vi "run_control.vi"() -> ()   [LabVIEW 2011]
uses:
  Dependencies/global.vi
panel:
  out "# of data":i32
  out "Real-time Data from Weather Station":string[][](array[string])
  out "Username":string
  out "Last Received Request":string
  in  "stop":bool
  out "Someone Connected?":bool
  out "Req / Res Error":errorcluster
  out "Remote Port":i64
  out "Remote Address":string
  out "Connection Error":errorcluster
  out "Real-time Data from PLCs (Actuation)":string[][](array[string])
  out "# of data":i32
  out "# of data":i32
  out "# of data":i32
  out "# of data":i32
  out "# of received data":u64
  out "Real-time Data from People Counter":string[][](array[string])
  out "Real-time Data from PLCs (Sensing)":string[][](array[string])
  out "Real-time Data from Motes":string[][](array[string])
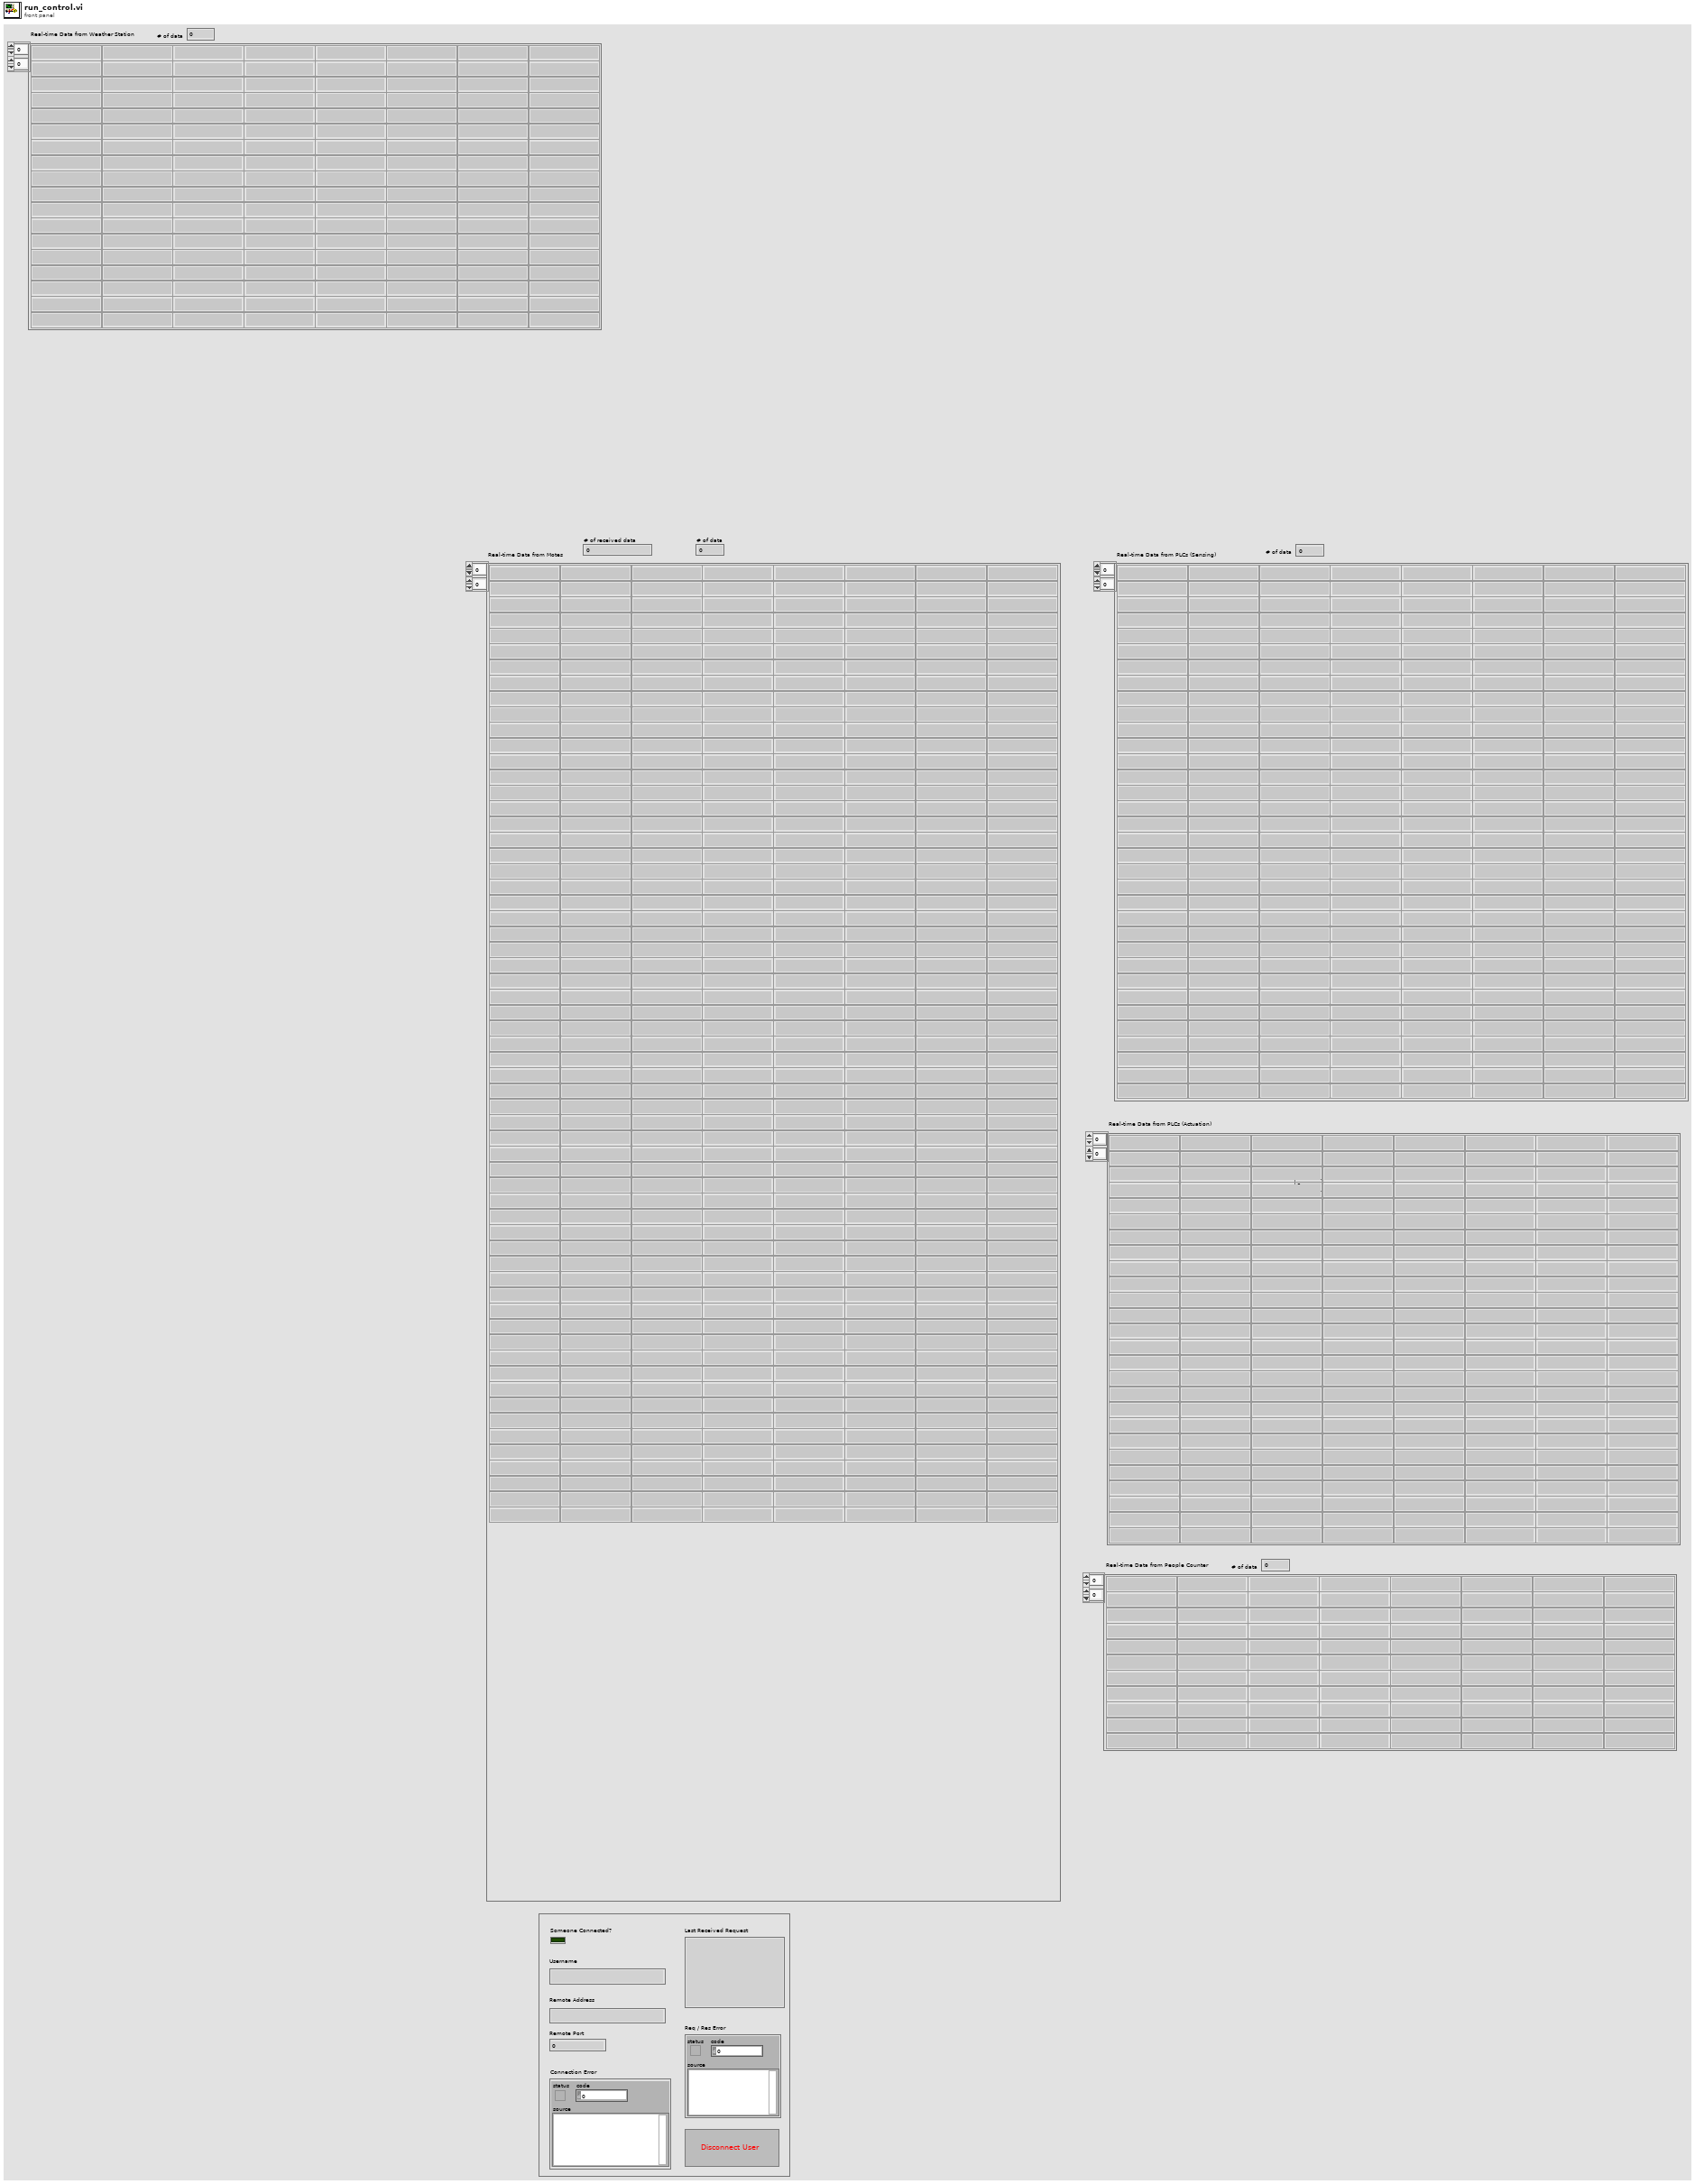
[diagram p1: front panel]
types:
  T1 = cluster{string, string, string, string, string, string, string, string}
  T2 = enum16{"Read", "Write", "ReadWrite", "BufferedRead", "BufferedReadWrite"}
  T3 = typedef "LVDateTimeRec.ctl" = cluster{"fractional second":dbl, "second":i32, "minute":i32, "hour":i32, "day of month":i32, "month":i32, "year":i32, "day of week":i32, "day of year":i32, "DST":i32}
  T4 = cluster{string, string, string, string, string, "date/time string":string, "output string":string, string}
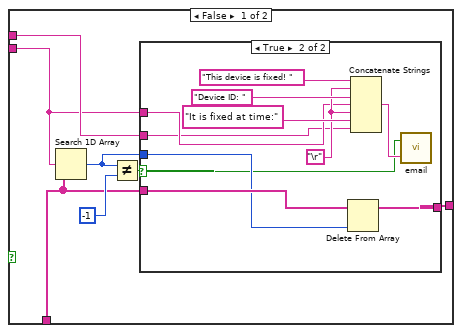
[diagram p3: hidden frame]
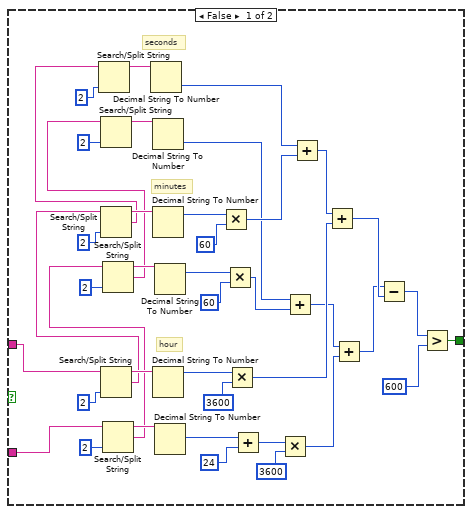
[diagram p6: hidden frame]
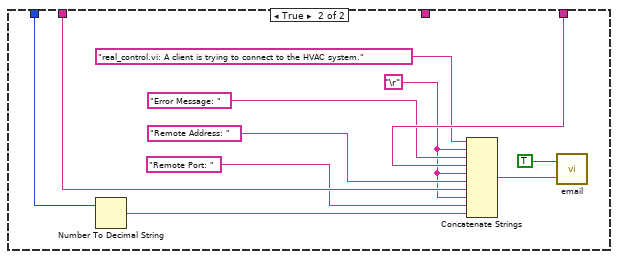
[diagram p7: hidden frame]
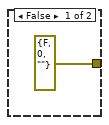
[diagram p8: hidden frame]
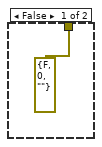
[diagram p9: hidden frame]
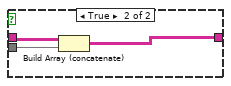
[diagram p10: hidden frame]
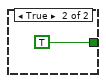
[diagram p11: hidden frame]
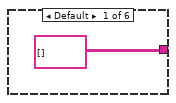
[diagram p12: hidden frame]
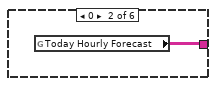
[diagram p13: hidden frame]
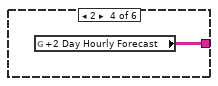
[diagram p14: hidden frame]
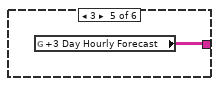
[diagram p15: hidden frame]
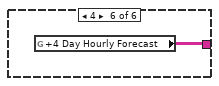
[diagram p16: hidden frame]
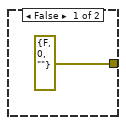
[diagram p17: hidden frame]
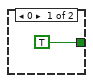
[diagram p18: hidden frame]
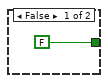
[diagram p19: hidden frame]
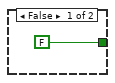
[diagram p20: hidden frame]
diagram:
  w1 = string[][] [["sourceType", "deviceID", "dataType", "signalID", "value", "timeStamp", "location", "coordinate"]] ("array")
  # "Real-time control Server"
  # "getting real-time data from database.vi"
  n1 = Bundle("", "", "", "", "", "", "", "") -> (w6:T1)  [unwired: 1 in]
  n2 = Obtain Queue(name (unnamed)="realtimeQue", element data type=w6) -> (queue out=w25:refnum<queue>)  [unwired: 3 in, 2 out]
  n3 = while {
    tunnel: w25 -> [w94]
    shift-right: [w41] -> _
    shift-left: w1 -> [w31]
    shift-right: [w40] -> _
    shift-left: w1 -> [w90]
    shift-right: [w79] -> _
    shift-left: w1 -> [w87]
    shift-right: [w42] -> _
    shift-left: w1 -> [w59]
    shift-right: [w29] -> _
    shift-left: w1 -> [w28]
    i -> [w86]
    stop <- TRUE continue-if-true
    n4 = Dequeue Element(queue=w94) -> (element=w44:T1)  [unwired: 2 in, 3 out]
    n5 = call "CommaToDot.vi"("Input"=w44) -> ("Output"=w30:T1)
    n6 = Unbundle(w30) -> (w33:string, w32:string, w27:string)  [unwired: 5 out]
    n7 = Unbundle(w30) -> (w55:string, w50:string, w49:string, w58:string)  [unwired: 4 out]
    n8 = Unbundle(w30) -> (w56:string, w52:string, w51:string)  [unwired: 5 out]
    n9 = Unbundle(w30) -> (w53:string, w46:string, w45:string)  [unwired: 5 out]
    n10 = Unbundle(w30) -> (w54:string, w48:string, w47:string, w57:string)  [unwired: 4 out]
    n11 = Equal?(x="6", y=w33) -> (x = y?=w39:bool)
    n12 = Not Equal?(x="A", y=w50) -> (x != y?=w71:bool)
    n13 = Equal?(x="2", y=w55) -> (x = y?=w70:bool)
    n14 = Equal?(x="A", y=w48) -> (x = y?=w66:bool)
    n15 = Equal?(x="2", y=w54) -> (x = y?=w67:bool)
    n16 = Equal?(x="1", y=w56) -> (x = y?=w92:bool)
    n17 = Equal?(x="3", y=w53) -> (x = y?=w89:bool)
    n18 = And(x=w71, y=w70) -> (x .and. y?=w69:bool)
    n19 = And(x=w66, y=w67) -> (x .and. y?=w68:bool)
    n20 = case shown="True" w39 {
      tunnel: w30 -> [_ w104]
      tunnel: w28 -> [w96 w98]
      tunnel: [w96 w99] -> w29
      tunnel: w32 -> [_ w103]
      tunnel: w27 -> [_ w97]
      frame False {
      }
      frame True {
        # "update array or add a new entry"
        # "search current array to see if the new data is already exists or not"
        n21 = for {
          tunnel: w98 -> [w116] mode=indexing
          tunnel: w103 -> [w119]
          tunnel: [w114] -> w102
          tunnel: [w118] -> w101
          tunnel: w97 -> [w115]
          i -> [w118]
          stop <- w114 stop-if-true
          # "key for weather station: deviceID and signalID"
          n22 = Index Array(array=w116, index=1) -> (element=w120:string)
          n23 = Equal?(x=w119, y=w120) -> (x = y?=w117:bool)
          n24 = case shown="True" w117 {
            tunnel: w116 -> [_ w126]
            tunnel: w115 -> [_ w124]
            tunnel: [FALSE w123] -> w114
            frame False {
            }
            frame True {
              n25 = Index Array(array=w126, index=3) -> (element=w125:string)
              n26 = Equal?(x=w124, y=w125) -> (x = y?=w123:bool)
            }
          }
        }
        n27 = Cluster To Array(cluster=w104) -> (array=w100:string[])
        n28 = case shown="True" w102 {
          tunnel: w98 -> [w109 w111]
          tunnel: w101 -> [w106 w110]
          tunnel: w100 -> [w108 w112]
          tunnel: [w107 w113] -> w99
          frame False {
            n29 = Increment(x=w106) -> (x+1=w105:i32)
            n30 = Insert Into Array(array=w109, index (row)=w105, new element=w108) -> (w107:string[][])  [unwired: 1 in]
          }
          frame True {
            n31 = Replace Array Subset(array=w111, new element=w112, index (row)=w110) -> (w113:string[][])  [unwired: 1 in]
          }
        }
      }
    }
    "Real-time Data from Weather Station" <- w29
    n32 = case shown="False" w69 {
      tunnel: w30 -> [_ w200]
      tunnel: w90 -> [w192 w195]
      tunnel: [w192 w196] -> w40
      tunnel: w49 -> [_ w194]
      tunnel: w58 -> [_ w193]
      frame False {
      }
      frame True {
        # "search current array to see if the new data is already exists or not"
        # "update array or add a new entry"
        n33 = for {
          tunnel: w195 -> [w211] mode=indexing
          tunnel: w194 -> [w215]
          tunnel: [w210] -> w199
          tunnel: [w214] -> w198
          tunnel: w193 -> [w212]
          i -> [w214]
          stop <- w210 stop-if-true
          # "key for plcs: signalID and location"
          n34 = Index Array(array=w211, index=3) -> (element=w216:string)
          n35 = Equal?(x=w215, y=w216) -> (x = y?=w213:bool)
          n36 = case shown="True" w213 {
            tunnel: w211 -> [_ w222]
            tunnel: w212 -> [_ w220]
            tunnel: [FALSE w219] -> w210
            frame False {
            }
            frame True {
              n37 = Index Array(array=w222, index=6) -> (element=w221:string)
              n38 = Equal?(x=w220, y=w221) -> (x = y?=w219:bool)
            }
          }
        }
        n39 = Cluster To Array(cluster=w200) -> (array=w197:string[])
        n40 = case shown="True" w199 {
          tunnel: w195 -> [w205 w207]
          tunnel: w198 -> [w202 w206]
          tunnel: w197 -> [w204 w208]
          tunnel: [w203 w209] -> w196
          frame False {
            n41 = Increment(x=w202) -> (x+1=w201:i32)
            n42 = Insert Into Array(array=w205, index (row)=w201, new element=w204) -> (w203:string[][])  [unwired: 1 in]
          }
          frame True {
            n43 = Replace Array Subset(array=w207, new element=w208, index (row)=w206) -> (w209:string[][])  [unwired: 1 in]
          }
        }
      }
    }
    "Real-time Data from PLCs (Sensing)" <- w40
    n44 = case shown="True" w92 {
      tunnel: w30 -> [_ w232]
      tunnel: w31 -> [w224 w226]
      tunnel: [w224 w227] -> w41
      tunnel: w52 -> [_ w231]
      tunnel: w51 -> [_ w225]
      frame False {
      }
      frame True {
        # "update array or add a new entry"
        # "search current array to see if the new data is already exists or not"
        n45 = for {
          tunnel: w226 -> [w244] mode=indexing
          tunnel: w231 -> [w247]
          tunnel: [w242] -> w230
          tunnel: [w246] -> w229
          tunnel: w225 -> [w243]
          i -> [w246]
          stop <- w242 stop-if-true
          # "key for motes: deviceID and dataType"
          n46 = Index Array(array=w244, index=1) -> (element=w248:string)
          n47 = Equal?(x=w247, y=w248) -> (x = y?=w245:bool)
          n48 = case shown="True" w245 {
            tunnel: w244 -> [_ w254]
            tunnel: w243 -> [_ w252]
            tunnel: [FALSE w251] -> w242
            frame False {
            }
            frame True {
              n49 = Index Array(array=w254, index=2) -> (element=w253:string)
              n50 = Equal?(x=w252, y=w253) -> (x = y?=w251:bool)
            }
          }
        }
        n51 = Cluster To Array(cluster=w232) -> (array=w228:string[])
        n52 = case shown="True" w230 {
          tunnel: w226 -> [w237 w239]
          tunnel: w229 -> [w234 w238]
          tunnel: w228 -> [w236 w240]
          tunnel: [w235 w241] -> w227
          frame False {
            n53 = Increment(x=w234) -> (x+1=w233:i32)
            n54 = Insert Into Array(array=w237, index (row)=w233, new element=w236) -> (w235:string[][])  [unwired: 1 in]
          }
          frame True {
            n55 = Replace Array Subset(array=w239, new element=w240, index (row)=w238) -> (w241:string[][])  [unwired: 1 in]
          }
        }
      }
    }
    "Real-time Data from Motes" <- w41
    n56 = case shown="True" w89 {
      tunnel: w30 -> [_ w168]
      tunnel: w87 -> [w160 w162]
      tunnel: [w160 w163] -> w79
      tunnel: w46 -> [_ w167]
      tunnel: w45 -> [_ w161]
      frame False {
      }
      frame True {
        # "update array or add a new entry"
        # "search current array to see if the new data is already exists or not"
        n57 = for {
          tunnel: w162 -> [w180] mode=indexing
          tunnel: w167 -> [w183]
          tunnel: [w178] -> w166
          tunnel: [w182] -> w165
          tunnel: w161 -> [w179]
          i -> [w182]
          stop <- w178 stop-if-true
          # "key for counter: deviceID and dataType"
          n58 = Index Array(array=w180, index=1) -> (element=w184:string)
          n59 = Equal?(x=w183, y=w184) -> (x = y?=w181:bool)
          n60 = case shown="True" w181 {
            tunnel: w180 -> [_ w190]
            tunnel: w179 -> [_ w188]
            tunnel: [FALSE w187] -> w178
            frame False {
            }
            frame True {
              n61 = Index Array(array=w190, index=2) -> (element=w189:string)
              n62 = Equal?(x=w188, y=w189) -> (x = y?=w187:bool)
            }
          }
        }
        n63 = Cluster To Array(cluster=w168) -> (array=w164:string[])
        n64 = case shown="True" w166 {
          tunnel: w162 -> [w173 w175]
          tunnel: w165 -> [w170 w174]
          tunnel: w164 -> [w172 w176]
          tunnel: [w171 w177] -> w163
          frame False {
            n65 = Increment(x=w170) -> (x+1=w169:i32)
            n66 = Insert Into Array(array=w173, index (row)=w169, new element=w172) -> (w171:string[][])  [unwired: 1 in]
          }
          frame True {
            n67 = Replace Array Subset(array=w175, new element=w176, index (row)=w174) -> (w177:string[][])  [unwired: 1 in]
          }
        }
      }
    }
    "Real-time Data from People Counter" <- w79
    n68 = case shown="True" w68 {
      tunnel: w30 -> [_ w136]
      tunnel: w59 -> [w128 w131]
      tunnel: [w128 w132] -> w42
      tunnel: w47 -> [_ w130]
      tunnel: w57 -> [_ w129]
      frame False {
      }
      frame True {
        # "search current array to see if the new data is already exists or not"
        # "update array or add a new entry"
        n69 = for {
          tunnel: w131 -> [w147] mode=indexing
          tunnel: w130 -> [w151]
          tunnel: [w146] -> w135
          tunnel: [w150] -> w134
          tunnel: w129 -> [w148]
          i -> [w150]
          stop <- w146 stop-if-true
          # "key for plcs: signalID and location"
          n70 = Index Array(array=w147, index=3) -> (element=w152:string)
          n71 = Equal?(x=w151, y=w152) -> (x = y?=w149:bool)
          n72 = case shown="True" w149 {
            tunnel: w147 -> [_ w158]
            tunnel: w148 -> [_ w156]
            tunnel: [FALSE w155] -> w146
            frame False {
            }
            frame True {
              n73 = Index Array(array=w158, index=6) -> (element=w157:string)
              n74 = Equal?(x=w156, y=w157) -> (x = y?=w155:bool)
            }
          }
        }
        n75 = Cluster To Array(cluster=w136) -> (array=w133:string[])
        n76 = case shown="False" w135 {
          tunnel: w131 -> [w141 w143]
          tunnel: w134 -> [w138 w142]
          tunnel: w133 -> [w140 w144]
          tunnel: [w139 w145] -> w132
          frame False {
            n77 = Increment(x=w138) -> (x+1=w137:i32)
            n78 = Insert Into Array(array=w141, index (row)=w137, new element=w140) -> (w139:string[][])  [unwired: 1 in]
          }
          frame True {
            n79 = Replace Array Subset(array=w143, new element=w144, index (row)=w142) -> (w145:string[][])  [unwired: 1 in]
          }
        }
      }
    }
    "Real-time Data from PLCs (Actuation)" <- w42
    n80 = Array Size(array=w29) -> (size(s)=w36:i32[])
    n81 = Array Size(array=w79) -> (size(s)=w80:i32[])
    n82 = Array Size(array=w41) -> (size(s)=w82:i32[])
    n83 = global write "global.vi" "Motes"(w41) -> ()
    n84 = global write "global.vi" "PLC Sensing"(w40) -> ()
    n85 = Array Size(array=w40) -> (size(s)=w85:i32[])
    n86 = Array Size(array=w42) -> (size(s)=w61:i32[])
    n87 = Index Array(array=w40, index (row)=1) -> ()  [unwired: 1 in, 1 out]
    n88 = global write "global.vi" "Actuation PLC"(w42) -> ()
    n89 = Index Array(array=w36, index=0) -> (element=w35:i32)
    n90 = Index Array(array=w80, index=0) -> (element=w74:i32)
    n91 = Index Array(array=w82, index=0) -> (element=w78:i32)
    n92 = Index Array(array=w85, index=0) -> (element=w76:i32)
    n93 = Index Array(array=w61, index=0) -> (element=w63:i32)
    n94 = Decrement(x=w35) -> (x-1=→"# of data":i32)
    n95 = Decrement(x=w78) -> (x-1=→"# of data":i32)
    n96 = Decrement(x=w74) -> (x-1=→"# of data":i32)
    n97 = Decrement(x=w76) -> (x-1=→"# of data":i32)
    n98 = Decrement(x=w63) -> (x-1=→"# of data":i32)
    "# of received data" <- w86
  }
  n99 = while {
    i -> [w258]
    stop <- TRUE continue-if-true
    n100 = local read "Real-time Data from PLCs (Actuation)"() -> (w257:string[][])
    n101 = local read "Real-time Data from Weather Station"() -> (w256:string[][])
    n102 = local read "Real-time Data from Motes"() -> (w260:string[][])
    n103 = call "writegraph.vi"("FromWeatherStation"=w256, "FromPLC"=w257, "Numeric"=w258, "FromMotes"=w260) -> ()  [unwired: 2 in]
    n104 = Wait (ms)(milliseconds to wait=u32 60000) -> ()  [unwired: 1 out]
  }
  n105 = Wait (ms)(milliseconds to wait=u32 30000) -> (millisecond timer value=w2:u32)
  n106 = flat-sequence {
    tunnel: w2 -> [_]
    frame #0 {
      n107 = while {
        shift-right: [w264] -> _
        shift-left: string[] [] ("Array") -> [w265]
        stop <- TRUE continue-if-true
        n108 = local read "# of data"() -> (w263:i32)
        n109 = Format Date/Time String(time format string (%c)="%y%m%d%H%M%S") -> (date/time string=w266:string)  [unwired: 2 in]
        n110 = for {
          N: w263 -> [_]
          tunnel: w266 -> [w288]
          shift-right: [w270] -> w264
          shift-left: w265 -> [w271]
          i -> [w296]
          # "same month?"
          # "same year?"
          n111 = Increment(x=w296) -> (x+1=w295:i32)
          n112 = Search/Split String(string=w288, offset (0)=2) -> (substring before match=w290:string, match + rest of string=w281:string)  [unwired: 1 in, 1 out]
          n113 = Search/Split String(string=w281, offset (0)=2) -> (substring before match=w283:string, match + rest of string=w274:string)  [unwired: 1 in, 1 out]
          n114 = local read "Real-time Data from Motes"() -> (w294:string[][])
          n115 = Decimal String To Number(string=w283) -> (number=w279:i32)  [unwired: 2 in, 1 out]
          n116 = Decimal String To Number(string=w290) -> (number=w289:i32)  [unwired: 2 in, 1 out]
          n117 = Index Array(array=w294, index (row)=w295, index (col)=1 ("disabled index (col)")) -> (element=w272:string)
          n118 = Index Array(array=w294, index (row)=w295, index (col)=5 ("disabled index (col)")) -> (element=w273:string)
          n119 = Search/Split String(string=w273, offset (0)=2) -> (substring before match=w292:string, match + rest of string=w282:string)  [unwired: 1 in, 1 out]
          n120 = Search/Split String(string=w282, offset (0)=2) -> (substring before match=w285:string, match + rest of string=w275:string)  [unwired: 1 in, 1 out]
          n121 = Decimal String To Number(string=w285) -> (number=w280:i32)  [unwired: 2 in, 1 out]
          n122 = Decimal String To Number(string=w292) -> (number=w287:i32)  [unwired: 2 in, 1 out]
          n123 = Equal?(x=w280, y=w279) -> (x = y?=w278:bool)
          n124 = Equal?(x=w287, y=w289) -> (x = y?=w277:bool)
          n125 = And(x=w277, y=w278) -> (x .and. y?=w276:bool)
          n126 = case shown="True" w276 {
            tunnel: w275 -> [_ w311]
            tunnel: w274 -> [_ w310]
            tunnel: w273 -> [_ w303]
            tunnel: w272 -> [_ w302]
            tunnel: w271 -> [w299 w301]
            tunnel: [w299 w300] -> w270
            frame False {
            }
            frame True {
              # "same day?"
              n127 = Search/Split String(string=w311, offset (0)=2) -> (substring before match=w314:string, match + rest of string=w306:string)  [unwired: 1 in, 1 out]
              n128 = Search/Split String(string=w310, offset (0)=2) -> (substring before match=w312:string, match + rest of string=w305:string)  [unwired: 1 in, 1 out]
              n129 = Decimal String To Number(string=w314) -> (number=w309:i32)  [unwired: 2 in, 1 out]
              n130 = Decimal String To Number(string=w312) -> (number=w308:i32)  [unwired: 2 in, 1 out]
              n131 = Equal?(x=w309, y=w308) -> (x = y?=w307:bool)
              n132 = case shown="True" w307 {
                tunnel: w306 -> [w357 w426]
                tunnel: w305 -> [w356 w425]
                tunnel: [w351 w392] -> w304
                frame False {
                  # "hour"
                  # "minutes"
                  # "seconds"
                  n133 = Search/Split String(string=w357, offset (0)=2) -> (substring before match=w390:string, match + rest of string=w383:string)  [unwired: 1 in, 1 out]
                  n134 = Search/Split String(string=w383, offset (0)=2) -> (substring before match=w386:string, match + rest of string=w377:string)  [unwired: 1 in, 1 out]
                  n135 = Search/Split String(string=w377, offset (0)=2) -> (substring before match=w380:string)  [unwired: 1 in, 2 out]
                  n136 = Search/Split String(string=w356, offset (0)=2) -> (substring before match=w388:string, match + rest of string=w382:string)  [unwired: 1 in, 1 out]
                  n137 = Search/Split String(string=w382, offset (0)=2) -> (substring before match=w384:string, match + rest of string=w376:string)  [unwired: 1 in, 1 out]
                  n138 = Search/Split String(string=w376, offset (0)=2) -> (substring before match=w378:string)  [unwired: 1 in, 2 out]
                  n139 = Decimal String To Number(string=w380) -> (number=w368:i32)  [unwired: 2 in, 1 out]
                  n140 = Decimal String To Number(string=w378) -> (number=w364:i32)  [unwired: 2 in, 1 out]
                  n141 = Decimal String To Number(string=w386) -> (number=w375:i32)  [unwired: 2 in, 1 out]
                  n142 = Decimal String To Number(string=w390) -> (number=w370:i32)  [unwired: 2 in, 1 out]
                  n143 = Decimal String To Number(string=w384) -> (number=w372:i32)  [unwired: 2 in, 1 out]
                  n144 = Decimal String To Number(string=w388) -> (number=w354:i32)  [unwired: 2 in, 1 out]
                  n145 = Multiply(x=w375, y=60) -> (x*y=w367:i32)
                  n146 = Multiply(x=w372, y=60) -> (x*y=w363:i32)
                  n147 = Multiply(x=w370, y=3600) -> (x*y=w365:i32)
                  n148 = Add(x=w354, y=24) -> (x+y=w353:i32)
                  n149 = Multiply(x=w353, y=3600) -> (x*y=w352:i32)
                  n150 = Add(x=w364, y=w363) -> (x+y=w362:i32)
                  n151 = Add(x=w368, y=w367) -> (x+y=w366:i32)
                  n152 = Add(x=w366, y=w365) -> (x+y=w361:i32)
                  n153 = Add(x=w362, y=w352) -> (x+y=w360:i32)
                  n154 = Subtract(x=w360, y=w361) -> (x-y=w359:i32)
                  n155 = Greater?(x=w359, y=600) -> (0:w351:bool)
                }
                frame True {
                  # "hour"
                  # "minutes"
                  # "seconds"
                  n156 = Search/Split String(string=w426, offset (0)=2) -> (substring before match=w429:string, match + rest of string=w420:string)  [unwired: 1 in, 1 out]
                  n157 = Search/Split String(string=w420, offset (0)=2) -> (substring before match=w423:string, match + rest of string=w414:string)  [unwired: 1 in, 1 out]
                  n158 = Search/Split String(string=w414, offset (0)=2) -> (substring before match=w417:string)  [unwired: 1 in, 2 out]
                  n159 = Search/Split String(string=w425, offset (0)=2) -> (substring before match=w427:string, match + rest of string=w419:string)  [unwired: 1 in, 1 out]
                  n160 = Search/Split String(string=w419, offset (0)=2) -> (substring before match=w421:string, match + rest of string=w413:string)  [unwired: 1 in, 1 out]
                  n161 = Search/Split String(string=w413, offset (0)=2) -> (substring before match=w415:string)  [unwired: 1 in, 2 out]
                  n162 = Decimal String To Number(string=w417) -> (number=w404:i32)  [unwired: 2 in, 1 out]
                  n163 = Decimal String To Number(string=w415) -> (number=w400:i32)  [unwired: 2 in, 1 out]
                  n164 = Decimal String To Number(string=w423) -> (number=w412:i32)  [unwired: 2 in, 1 out]
                  n165 = Decimal String To Number(string=w429) -> (number=w407:i32)  [unwired: 2 in, 1 out]
                  n166 = Decimal String To Number(string=w421) -> (number=w409:i32)  [unwired: 2 in, 1 out]
                  n167 = Decimal String To Number(string=w427) -> (number=w405:i32)  [unwired: 2 in, 1 out]
                  n168 = Multiply(x=w412, y=60) -> (x*y=w403:i32)
                  n169 = Multiply(x=w409, y=60) -> (x*y=w399:i32)
                  n170 = Multiply(x=w407, y=3600) -> (x*y=w401:i32)
                  n171 = Multiply(x=w405, y=3600) -> (x*y=w397:i32)
                  n172 = Add(x=w400, y=w399) -> (x+y=w398:i32)
                  n173 = Add(x=w404, y=w403) -> (x+y=w402:i32)
                  n174 = Add(x=w402, y=w401) -> (x+y=w396:i32)
                  n175 = Add(x=w398, y=w397) -> (x+y=w395:i32)
                  n176 = Subtract(x=w395, y=w396) -> (x-y=w394:i32)
                  n177 = Greater?(x=w394, y=600) -> (0:w392:bool)
                }
              }
              n178 = case shown="True" w304 {
                tunnel: w302 -> [w316 w335]
                tunnel: w303 -> [w317 w339]
                tunnel: w301 -> [w320 w338]
                tunnel: [w318 w337] -> w300
                frame False {
                  n179 = Search 1D Array(1D array=w320, element=w316) -> (index of element=w319:i32)  [unwired: 1 in]
                  n180 = Not Equal?(x=w319, y=-1) -> (x != y?=w321:bool)
                  n181 = case shown="True" w321 {
                    selector: w321 -> [_ w326]
                    tunnel: w320 -> [w323 w334]
                    tunnel: w319 -> [_ w329]
                    tunnel: [w323 w333] -> w318
                    tunnel: w316 -> [_ w325]
                    tunnel: w317 -> [_ w324]
                    frame False {
                    }
                    frame True {
                      w328 = "\r"
                      n182 = Delete From Array(array=w334, index=w329) -> (array with subset deleted=w333:string[])  [unwired: 1 in, 1 out]
                      n183 = Concatenate Strings("This device is fixed! " ("string"), w328, "Device ID: " ("string"), w325, w328, "It is fixed at time:" ("string"), w324) -> (w327:string)
                      n184 = call "email.vi"("Body"=w327, "Enable"=w326) -> ()  [unwired: 1 in]
                    }
                  }
                }
                frame True {
                  w344 = "\r"
                  n185 = Search 1D Array(1D array=w338, element=w335) -> (index of element=w341:i32)  [unwired: 1 in]
                  n186 = Equal?(x=w341, y=-1) -> (x = y?=w336:bool)
                  n187 = case shown="True" w336 {
                    tunnel: w338 -> [w347 w350]
                    tunnel: [w347 w349] -> w337
                    tunnel: w335 -> [_ w348]
                    frame False {
                    }
                    frame True {
                      n188 = Insert Into Array(array=w350, new element=w348) -> (w349:string[])  [unwired: 1 in]
                    }
                  }
                  n189 = Concatenate Strings("This device is not working! " ("string"), w344, "Device ID: " ("string"), w335, w344, "No data received from this mote since time:" ("string"), w339) -> (w342:string)
                  n190 = call "email.vi"("Body"=w342, "Enable"=w336) -> ()  [unwired: 1 in]
                }
              }
            }
          }
        }
        n191 = Wait (ms)(milliseconds to wait=u32 30000) -> ()  [unwired: 1 out]
      }
    }
  }
  n192 = Bundle("", "", "", "", "", "", "", "") -> (w20:T1)  [unwired: 1 in]
  n193 = Obtain Queue(max queue size (-1, unlimited)=-1, name (unnamed)="databaseQue", element data type=w20) -> (queue out=w15:refnum<queue>)  [unwired: 2 in, 2 out]
  n194 = while {
    tunnel: w15 -> [w439]
    stop <- TRUE continue-if-true
    n195 = call <vilib>:"TCP Listen.vi"("port"=u16 6342) -> ("error out"=w434:errorcluster, "remote port"=w432:u16, "remote address"=w433:string, "connection ID"=w435:refnum<k5>)  [unwired: 6 in, 1 out]
    "Remote Address" <- w433
    "Remote Port" <- w432
    n196 = local write "Someone Connected?"(FALSE ("Someone Connected?")) -> ()
    n197 = call "credentialCheck.vi"("connection ID in"=w435, "error in"=w434) -> ("connection ID out"=w442:refnum<k5>, "user"=w437:string, "error out"=w441:errorcluster)
    "Connection Error" <- w441
    "Username" <- w437
    n198 = Unbundle(w441) -> ("status"=w438:bool, "source"=w440:string)  [unwired: 1 out]
    n199 = case shown="False" w438 {
      tunnel: w432 -> [w445 w463]
      tunnel: w440 -> [_ w462]
      tunnel: w433 -> [w446 w458]
      tunnel: w437 -> [w444 _]
      frame False {
        w449 = "\r"
        n200 = Number To Decimal String(number=w445) -> (decimal integer string=w447:string)  [unwired: 1 in]
        n201 = Concatenate Strings("real_control.vi: A client connected to the HVAC system.", w449, "Username: ", w444, w449, "Remote Address: ", w446, w449, "Remote Port: ", w447) -> (w454:string)
        n202 = call "email.vi"("Body"=w454, "Enable"=FALSE) -> ()  [unwired: 1 in]
      }
      frame True {
        w457 = "\r"
        n203 = Number To Decimal String(number=w463) -> (decimal integer string=w455:string)  [unwired: 1 in]
        n204 = Concatenate Strings("real_control.vi: A client is trying to connect to the HVAC system.", w457, "Error Message: ", w462, w457, "Remote Address: ", w458, w457, "Remote Port: ", w455) -> (w465:string)
        n205 = call "email.vi"("Body"=w465, "Enable"=TRUE) -> ()  [unwired: 1 in]
      }
    }
    n206 = case shown="No Error" w441 {
      tunnel: w442 -> [w467 _]
      tunnel: w439 -> [w466 _]
      frame No Error {
        n207 = while {
          tunnel: w467 -> [w536]
          tunnel: w466 -> [w493]
          stop <- w475 stop-if-true
          # "signalID"
          # "To hour"
          # "From hour"
          # "signalID"
          # "deviceID"
          # "dataType"
          # "data"
          # "stop the loop if any problem\noccures in the TCP blocks. Normally\nit means the client terminated the\nconnection."
          # "location"
          # "signalID"
          # "dataType"
          # "deviceID"
          # "Then read all input \nparameters from client"
          # "signalID"
          # "dataType"
          # "deviceID"
          # "first read the size of input \nparameters from client"
          n208 = TCP Read(connection ID=w536, bytes to read=10, 9:-1 ("timeout ms (25000)")) -> (connection ID out=w532:refnum<k5>, data out=w533:string, error out=w531:errorcluster)  [unwired: 2 in]
          n209 = local write "Someone Connected?"(TRUE ("Someone Connected?")) -> ()
          n210 = Decimal String To Number(string=w533) -> (number=w530:i32)  [unwired: 2 in, 1 out]
          n211 = TCP Read(connection ID=w532, bytes to read=w530, error in (no error)=w531) -> (connection ID out=w479:refnum<k5>, data out=w470:string, error out=w523:errorcluster)  [unwired: 2 in]
          "Last Received Request" <- w470
          n212 = Pick Line(multi-line string=w470, line index=2) -> (output string=w503:string)  [unwired: 1 in]
          n213 = Pick Line(multi-line string=w470, line index=1) -> (output string=w502:string)  [unwired: 1 in]
          n214 = Pick Line(multi-line string=w470, line index=3) -> (output string=w504:string)  [unwired: 1 in]
          n215 = Pick Line(multi-line string=w470, line index=0) -> (output string=w501:string)  [unwired: 1 in]
          n216 = Pick Line(multi-line string=w470, line index=0) -> (output string=w482:string)  [unwired: 1 in]
          n217 = Pick Line(multi-line string=w470, line index=1) -> (output string=w485:string)  [unwired: 1 in]
          n218 = Pick Line(multi-line string=w470, line index=0) -> (output string=w487:string)  [unwired: 1 in]
          n219 = Pick Line(multi-line string=w470, line index=2) -> (output string=w484:string)  [unwired: 1 in]
          n220 = Pick Line(multi-line string=w470, line index=2) -> (output string=w508:string)  [unwired: 1 in]
          n221 = Pick Line(multi-line string=w470, line index=1) -> (output string=w476:string)  [unwired: 1 in]
          n222 = Pick Line(multi-line string=w470, line index=3) -> (output string=w506:string)  [unwired: 1 in]
          n223 = Pick Line(multi-line string=w470, line index=0) -> (output string=w509:string)  [unwired: 1 in]
          n224 = Pick Line(multi-line string=w470, line index=2) -> (output string=w471:string)  [unwired: 1 in]
          n225 = Pick Line(multi-line string=w470, line index=1) -> (output string=w522:string)  [unwired: 1 in]
          n226 = Pick Line(multi-line string=w470, line index=3) -> (output string=w469:string)  [unwired: 1 in]
          n227 = Pick Line(multi-line string=w470, line index=0) -> (output string=w521:string)  [unwired: 1 in]
          n228 = Pick Line(multi-line string=w470, line index=2) -> (output string=w526:string)  [unwired: 1 in]
          n229 = Pick Line(multi-line string=w470, line index=1) -> (output string=w527:string)  [unwired: 1 in]
          n230 = Pick Line(multi-line string=w470, line index=3) -> (output string=w525:string)  [unwired: 1 in]
          n231 = Pick Line(multi-line string=w470, line index=0) -> (output string=w528:string)  [unwired: 1 in]
          n232 = Equal?(x="GetDataWeatherNow", y=w482) -> (x = y?=w483:bool)
          n233 = Equal?(x="GetDataPCounter", y=w501) -> (x = y?=w499:bool)
          n234 = Equal?(x="GetDataWeatherForecast", y=w487) -> (x = y?=w486:bool)
          n235 = Equal?(x="GetDataPlcs", y=w521) -> (x = y?=w519:bool)
          n236 = case shown="True" w499 {
            tunnel: w502 -> [_ w655]
            tunnel: w503 -> [_ w654]
            tunnel: w504 -> [_ w653]
            tunnel: w479 -> [_ w647]
            tunnel: [errorcluster {"status"=FALSE, "code"=0, "source"=""} ("error IO") w648] -> w494
            frame False {
            }
            frame True {
              # "check each row of the array to see if it matches. If yes, append that row to the result array"
              n237 = local read "Real-time Data from People Counter"() -> (w650:string[][])
              n238 = for {
                tunnel: w650 -> [w681] mode=indexing
                tunnel: w655 -> [w683]
                tunnel: w654 -> [w688]
                tunnel: w653 -> [w687]
                shift-right: [w685] -> w651
                shift-left: string[][] [] -> [w682]
                i -> [w680]
                stop <- TRUE continue-if-true
                n239 = case shown="Default" w680 {
                  tunnel: w688 -> [_ w698]
                  tunnel: w687 -> [_ w697]
                  tunnel: [TRUE w696] -> w686
                  tunnel: w683 -> [_ w695]
                  tunnel: w681 -> [_ w690]
                  frame 0 {
                  }
                  frame Default {
                    n240 = Index Array(array=w690, index=1) -> (element=w699:string)
                    n241 = Empty String/Path?(string/path=w695) -> (empty?=w693:bool)
                    n242 = Equal?(x=w695, y=w699) -> (x = y?=w694:bool)
                    n243 = Or(x=w693, y=w694) -> (x .or. y?=w692:bool)
                    n244 = case shown="True" w692 {
                      tunnel: w690 -> [_ w715]
                      tunnel: w698 -> [_ w710]
                      tunnel: [FALSE w713] -> w691
                      frame False {
                      }
                      frame True {
                        n245 = Index Array(array=w715, index=2) -> (element=w714:string)
                        n246 = Empty String/Path?(string/path=w710) -> (empty?=w711:bool)
                        n247 = Equal?(x=w710, y=w714) -> (x = y?=w712:bool)
                        n248 = Or(x=w711, y=w712) -> (x .or. y?=w713:bool)
                      }
                    }
                    n249 = case shown="True" w691 {
                      tunnel: w690 -> [_ w707]
                      tunnel: w697 -> [_ w703]
                      tunnel: [FALSE w702] -> w696
                      frame False {
                      }
                      frame True {
                        n250 = Index Array(array=w707, index=3) -> (element=w706:string)
                        n251 = Equal?(x=w703, y=w706) -> (x = y?=w705:bool)
                        n252 = Empty String/Path?(string/path=w703) -> (empty?=w704:bool)
                        n253 = Or(x=w704, y=w705) -> (x .or. y?=w702:bool)
                      }
                    }
                  }
                }
                n254 = case shown="True" w686 {
                  tunnel: w682 -> [w717 w720]
                  tunnel: w681 -> [_ w719]
                  tunnel: [w717 w718] -> w685
                  frame False {
                  }
                  frame True {
                    n255 = Build Array (concatenate)(w720, w719) -> (w718:string[][])
                  }
                }
              }
              n256 = flat-sequence {
                tunnel: w651 -> [w658]
                tunnel: w647 -> [w657]
                tunnel: [w656] -> w649
                tunnel: w649 -> [w672]
                tunnel: [w671] -> w648
                tunnel: w647 -> [w670]
                frame #0 {
                  # "send each element of the array through the TCP connection"
                  n257 = for {
                    tunnel: w658 -> [w661] mode=indexing
                    tunnel: w657 -> [w660]
                    tunnel: [w659] -> w656
                    n258 = for {
                      tunnel: w661 -> [w664] mode=indexing
                      tunnel: w660 -> [w663]
                      tunnel: [w662] -> w659
                      n259 = String Length(string=w664) -> (length=w668:i32)
                      n260 = Number To Decimal String(number=w668, width (-)=i16 10) -> (decimal integer string=w667:string)
                      n261 = TCP Write(connection ID=w663, data in=w667) -> (connection ID out=w665:refnum<k5>, error out=w666:errorcluster)  [unwired: 2 in, 1 out]
                      n262 = TCP Write(connection ID=w665, data in=w664, error in (no error)=w666) -> (error out=w662:errorcluster)  [unwired: 1 in, 2 out]
                    }
                  }
                }
                frame #1 {
                  w674 = "EndOfTx" ("data in")
                  n263 = String Length(string=w674) -> (length=w677:i32)
                  n264 = Number To Decimal String(number=w677, width (-)=i16 10) -> (decimal integer string=w678:string)
                  n265 = TCP Write(connection ID=w670, data in=w678) -> (connection ID out=w675:refnum<k5>, error out=w679:errorcluster)  [unwired: 2 in, 1 out]
                  n266 = TCP Write(connection ID=w675, data in=w674, error in (no error)=w679) -> (error out=w673:errorcluster)  [unwired: 1 in, 2 out]
                  n267 = Merge Errors(w673, w672) -> (w671:errorcluster)
                }
              }
            }
          }
          n268 = Equal?(x="SetDataPlcs", y=w509) -> (x = y?=w511:bool)
          n269 = case shown="True" w483 {
            tunnel: w479 -> [_ w545]
            tunnel: [errorcluster {"status"=FALSE, "code"=0, "source"=""} ("error IO") w544] -> w477
            frame False {
            }
            frame True {
              n270 = global read "global.vi" "Now"() -> (w543:string[][])
              n271 = flat-sequence {
                tunnel: w543 -> [w549]
                tunnel: w545 -> [w548]
                tunnel: [w547] -> w546
                tunnel: w546 -> [w563]
                tunnel: [w562] -> w544
                tunnel: w545 -> [w561]
                frame #0 {
                  # "send each element of the array through the TCP connection"
                  n272 = for {
                    tunnel: w549 -> [w552] mode=indexing
                    tunnel: w548 -> [w551]
                    tunnel: [w550] -> w547
                    n273 = for {
                      tunnel: w552 -> [w555] mode=indexing
                      tunnel: w551 -> [w554]
                      tunnel: [w553] -> w550
                      n274 = String Length(string=w555) -> (length=w559:i32)
                      n275 = Number To Decimal String(number=w559, width (-)=i16 10) -> (decimal integer string=w558:string)
                      n276 = TCP Write(connection ID=w554, data in=w558) -> (connection ID out=w556:refnum<k5>, error out=w557:errorcluster)  [unwired: 2 in, 1 out]
                      n277 = TCP Write(connection ID=w556, data in=w555, error in (no error)=w557) -> (error out=w553:errorcluster)  [unwired: 1 in, 2 out]
                    }
                  }
                }
                frame #1 {
                  w565 = "EndOfTx" ("data in")
                  n278 = String Length(string=w565) -> (length=w568:i32)
                  n279 = Number To Decimal String(number=w568, width (-)=i16 10) -> (decimal integer string=w569:string)
                  n280 = TCP Write(connection ID=w561, data in=w569) -> (connection ID out=w566:refnum<k5>, error out=w570:errorcluster)  [unwired: 2 in, 1 out]
                  n281 = TCP Write(connection ID=w566, data in=w565, error in (no error)=w570) -> (error out=w564:errorcluster)  [unwired: 1 in, 2 out]
                  n282 = Merge Errors(w564, w563) -> (w562:errorcluster)
                }
              }
            }
          }
          n283 = case shown="True" w486 {
            tunnel: w485 -> [_ w577]
            tunnel: w484 -> [_ w582]
            tunnel: w479 -> [_ w578]
            tunnel: [errorcluster {"status"=FALSE, "code"=0, "source"=""} ("error IO") w572] -> w478
            frame False {
            }
            frame True {
              n284 = Decimal String To Number(string=w577) -> (number=w575:i32)  [unwired: 2 in, 1 out]
              n285 = Decimal String To Number(string=w582) -> (number=w576:i32)  [unwired: 2 in, 1 out]
              n286 = Subtract(x=w576, y=w575) -> (x-y=w574:i32)
              n287 = Increment(x=w574) -> (x+1=w573:i32)
              n288 = for {
                N: w573 -> [_]
                shift-right: [w614] -> w579
                shift-left: string[][] [] -> [w616]
                shift-right: [w611] -> _
                shift-left: w575 -> [w610]
                i -> [w609]
                n289 = call "which_day.vi"("Hour"=w610) -> ("which array"=w618:i32, "New Date"=w617:T3)
                n290 = Increment(x=w610) -> (x+1=w611:i32)
                n291 = Unbundle(w617) -> ("hour"=w607:i32)  [unwired: 9 out]
                n292 = case shown="1" w618 {
                  tunnel: [string[][] [] w641 w642 w643 w644 w645] -> w613
                  frame Default {
                  }
                  frame 0 {
                    n293 = global read "global.vi" "Today Hourly Forecast"() -> (w641:string[][])
                  }
                  frame 1 {
                    n294 = global read "global.vi" "+1 Day Hourly Forecast"() -> (w642:string[][])
                  }
                  frame 2 {
                    n295 = global read "global.vi" "+2 Day Hourly Forecast"() -> (w643:string[][])
                  }
                  frame 3 {
                    n296 = global read "global.vi" "+3 Day Hourly Forecast"() -> (w644:string[][])
                  }
                  frame 4 {
                    n297 = global read "global.vi" "+4 Day Hourly Forecast"() -> (w645:string[][])
                  }
                }
                n298 = Equal To 0?(x=w609) -> (x = 0?=w608:bool)
                n299 = for {
                  tunnel: w613 -> [w625] mode=indexing
                  shift-right: [w624] -> w615
                  shift-left: string[][] [] -> [w626]
                  tunnel: w607 -> [w623]
                  tunnel: w608 -> [w620]
                  i -> [w622]
                  n300 = Equal To 0?(x=w622) -> (x = 0?=w621:bool)
                  n301 = And(x=w620, y=w621) -> (x .and. y?=w619:bool)
                  n302 = case shown="False" w619 {
                    tunnel: w625 -> [w637 _]
                    tunnel: [w636 TRUE] -> w627
                    tunnel: w623 -> [w635 _]
                    frame False {
                      n303 = Index Array(array=w637, index=4) -> (element=w634:string)
                      n304 = Decimal String To Number(string=w634, default (0L)=-1 ("default (0 I32)")) -> (number=w633:i32)  [unwired: 1 in, 1 out]
                      n305 = Equal?(x=w635, y=w633) -> (x = y?=w636:bool)
                    }
                    frame True {
                    }
                  }
                  n306 = case shown="False" w627 {
                    tunnel: w626 -> [w628 w631]
                    tunnel: w625 -> [_ w630]
                    tunnel: [w628 w629] -> w624
                    frame False {
                    }
                    frame True {
                      n307 = Build Array (concatenate)(w631, w630) -> (w629:string[][])
                    }
                  }
                }
                n308 = Build Array (concatenate)(w616, w615) -> (w614:string[][])
              }
              n309 = flat-sequence {
                tunnel: w579 -> [w585]
                tunnel: w578 -> [w584]
                tunnel: [w583] -> w580
                tunnel: w580 -> [w599]
                tunnel: [w598] -> w572
                tunnel: w578 -> [w597]
                frame #0 {
                  # "send each element of the array through the TCP connection"
                  n310 = for {
                    tunnel: w585 -> [w588] mode=indexing
                    tunnel: w584 -> [w587]
                    tunnel: [w586] -> w583
                    n311 = for {
                      tunnel: w588 -> [w591] mode=indexing
                      tunnel: w587 -> [w590]
                      tunnel: [w589] -> w586
                      n312 = String Length(string=w591) -> (length=w595:i32)
                      n313 = Number To Decimal String(number=w595, width (-)=i16 10) -> (decimal integer string=w594:string)
                      n314 = TCP Write(connection ID=w590, data in=w594) -> (connection ID out=w592:refnum<k5>, error out=w593:errorcluster)  [unwired: 2 in, 1 out]
                      n315 = TCP Write(connection ID=w592, data in=w591, error in (no error)=w593) -> (error out=w589:errorcluster)  [unwired: 1 in, 2 out]
                    }
                  }
                }
                frame #1 {
                  w601 = "EndOfTx" ("data in")
                  n316 = String Length(string=w601) -> (length=w604:i32)
                  n317 = Number To Decimal String(number=w604, width (-)=i16 10) -> (decimal integer string=w605:string)
                  n318 = TCP Write(connection ID=w597, data in=w605) -> (connection ID out=w602:refnum<k5>, error out=w606:errorcluster)  [unwired: 2 in, 1 out]
                  n319 = TCP Write(connection ID=w602, data in=w601, error in (no error)=w606) -> (error out=w600:errorcluster)  [unwired: 1 in, 2 out]
                  n320 = Merge Errors(w600, w599) -> (w598:errorcluster)
                }
              }
            }
          }
          n321 = case shown="True" w519 {
            tunnel: w522 -> [_ w888]
            tunnel: w471 -> [_ w887]
            tunnel: w479 -> [_ w891]
            tunnel: [errorcluster {"status"=FALSE, "code"=0, "source"=""} ("error IO") w893] -> w515
            tunnel: w469 -> [_ w886]
            frame False {
            }
            frame True {
              n322 = local read "Real-time Data from PLCs (Sensing)"() -> (w890:string[][])
              n323 = for {
                tunnel: w890 -> [w895] mode=indexing
                tunnel: w888 -> [w897]
                tunnel: w887 -> [w902]
                tunnel: w886 -> [w901]
                shift-right: [w899] -> w885
                shift-left: string[][] [] -> [w896]
                i -> [w894]
                stop <- TRUE continue-if-true
                n324 = case shown="Default" w894 {
                  tunnel: w902 -> [_ w915]
                  tunnel: w901 -> [_ w914]
                  tunnel: [TRUE w913] -> w900
                  tunnel: w897 -> [_ w912]
                  tunnel: w895 -> [_ w911]
                  tunnel: w895 -> [_ w904]
                  frame 0 {
                  }
                  frame Default {
                    n325 = Index Array(array=w911, index=1) -> (element=w909:string)
                    n326 = Empty String/Path?(string/path=w912) -> (empty?=w907:bool)
                    n327 = Equal?(x=w912, y=w909) -> (x = y?=w908:bool)
                    n328 = Or(x=w907, y=w908) -> (x .or. y?=w906:bool)
                    n329 = case shown="True" w906 {
                      tunnel: w911 -> [_ w930]
                      tunnel: w915 -> [_ w925]
                      tunnel: [FALSE w928] -> w905
                      frame False {
                      }
                      frame True {
                        n330 = Index Array(array=w930, index=2) -> (element=w929:string)
                        n331 = Empty String/Path?(string/path=w925) -> (empty?=w926:bool)
                        n332 = Equal?(x=w925, y=w929) -> (x = y?=w927:bool)
                        n333 = Or(x=w926, y=w927) -> (x .or. y?=w928:bool)
                      }
                    }
                    n334 = case shown="True" w905 {
                      tunnel: w904 -> [_ w922]
                      tunnel: w914 -> [_ w918]
                      tunnel: [FALSE w917] -> w913
                      frame False {
                      }
                      frame True {
                        n335 = Index Array(array=w922, index=3) -> (element=w921:string)
                        n336 = Equal?(x=w918, y=w921) -> (x = y?=w920:bool)
                        n337 = Empty String/Path?(string/path=w918) -> (empty?=w919:bool)
                        n338 = Or(x=w919, y=w920) -> (x .or. y?=w917:bool)
                      }
                    }
                  }
                }
                n339 = case shown="True" w900 {
                  tunnel: w896 -> [w932 w935]
                  tunnel: w895 -> [_ w934]
                  tunnel: [w932 w933] -> w899
                  frame False {
                  }
                  frame True {
                    n340 = Build Array (concatenate)(w935, w934) -> (w933:string[][])
                  }
                }
              }
              n341 = flat-sequence {
                tunnel: w885 -> [w938]
                tunnel: w891 -> [w937]
                tunnel: [w936] -> w892
                tunnel: [w952] -> w893
                tunnel: w892 -> [w951]
                tunnel: w891 -> [w950]
                frame #0 {
                  # "send each element of the array through the TCP connection"
                  n342 = for {
                    tunnel: w938 -> [w941] mode=indexing
                    tunnel: w937 -> [w940]
                    tunnel: [w939] -> w936
                    n343 = for {
                      tunnel: w941 -> [w944] mode=indexing
                      tunnel: w940 -> [w943]
                      tunnel: [w942] -> w939
                      n344 = String Length(string=w944) -> (length=w948:i32)
                      n345 = Number To Decimal String(number=w948, width (-)=i16 10) -> (decimal integer string=w947:string)
                      n346 = TCP Write(connection ID=w943, data in=w947) -> (connection ID out=w945:refnum<k5>, error out=w946:errorcluster)  [unwired: 2 in, 1 out]
                      n347 = TCP Write(connection ID=w945, data in=w944, error in (no error)=w946) -> (error out=w942:errorcluster)  [unwired: 1 in, 2 out]
                    }
                  }
                }
                frame #1 {
                  w954 = "EndOfTx" ("data in")
                  n348 = String Length(string=w954) -> (length=w957:i32)
                  n349 = Number To Decimal String(number=w957, width (-)=i16 10) -> (decimal integer string=w958:string)
                  n350 = TCP Write(connection ID=w950, data in=w958) -> (connection ID out=w955:refnum<k5>, error out=w959:errorcluster)  [unwired: 2 in, 1 out]
                  n351 = TCP Write(connection ID=w955, data in=w954, error in (no error)=w959) -> (error out=w953:errorcluster)  [unwired: 1 in, 2 out]
                  n352 = Merge Errors(w953, w951) -> (w952:errorcluster)
                }
              }
            }
          }
          n353 = Equal?(x="GetDataMotes", y=w528) -> (x = y?=w535:bool)
          n354 = case shown="True" w511 {
            tunnel: w476 -> [_ w763]
            tunnel: w508 -> [_ w762]
            tunnel: w479 -> [_ w761]
            tunnel: w479 -> [_ w741]
            tunnel: w508 -> [_ w724]
            tunnel: w476 -> [_ w723]
            tunnel: w506 -> [_ w728]
            tunnel: [errorcluster {"status"=FALSE, "code"=0, "source"=""} ("error IO") w727] -> w505
            tunnel: w493 -> [_ w725]
            frame False {
            }
            frame True {
              # "check to see if we can find the entry in the table. We should find only and only 1 entry!"
              n355 = local read "Real-time Data from PLCs (Actuation)"() -> (w760:string[][])
              n356 = for {
                tunnel: w760 -> [w863] mode=indexing
                tunnel: w763 -> [w867]
                tunnel: w762 -> [w870]
                shift-right: [w869] -> w742
                shift-left: u64 0 -> [w861]
                stop <- TRUE continue-if-true
                n357 = Index Array(array=w863, index=3) -> (element=w871:string)
                n358 = Empty String/Path?(string/path=w867) -> (empty?=w865:bool)
                n359 = Equal?(x=w867, y=w871) -> (x = y?=w866:bool)
                n360 = Or(x=w865, y=w866) -> (x .or. y?=w864:bool)
                n361 = case shown="True" w864 {
                  tunnel: w863 -> [_ w882]
                  tunnel: w870 -> [_ w877]
                  tunnel: [FALSE w880] -> w862
                  frame False {
                  }
                  frame True {
                    n362 = Index Array(array=w882, index=6) -> (element=w881:string)
                    n363 = Empty String/Path?(string/path=w877) -> (empty?=w878:bool)
                    n364 = Equal?(x=w877, y=w881) -> (x = y?=w879:bool)
                    n365 = Or(x=w878, y=w879) -> (x .or. y?=w880:bool)
                  }
                }
                n366 = case shown="True" w862 {
                  tunnel: [w873 w874] -> w869
                  tunnel: w861 -> [w873 w875]
                  frame False {
                  }
                  frame True {
                    n367 = Increment(x=w875) -> (x+1=w874:u64)
                  }
                }
              }
              n368 = case shown="\"65\"" w723 {
                tunnel: ["" "ST901" "ST902" "SV201" "SV401"] -> w722
                frame Default {
                }
                frame "61" {
                }
                frame "62" {
                }
                frame "63" {
                }
                frame "65" {
                }
              }
              n369 = Fract/Exp String To Number(string=w728) -> (number=w729:dbl)  [unwired: 3 in, 1 out]
              n370 = Fract/Exp String To Number(string=w728) -> (number=w735:dbl)  [unwired: 3 in, 1 out]
              n371 = Greater Or Equal?(x=w729, y=0.0) -> (x >= y?=w734:bool)
              n372 = Less Or Equal?(x=w729, y=100.0) -> (x <= y?=w733:bool)
              n373 = Greater Or Equal?(x=w735, y=0.0) -> (x >= y?=w737:bool)
              n374 = Less Or Equal?(x=w735, y=100.0) -> (x <= y?=w738:bool)
              n375 = And(x=w733, y=w734) -> (x .and. y?=w730:bool)
              n376 = Not And(1:w737, 2:w738) -> (0:w736:bool)
              n377 = Concatenate Strings("opc://localhost/Fidelix.FdxOPC/AS_KTH.AO.", w724, "_", w722, "_SF.Value") -> (w752:string)
              n378 = Equal?(x=w742, y=u64 1) -> (x = y?=w745:bool)
              n379 = Equal To 0?(x=w742) -> (x = 0?=w758:bool)
              n380 = Equal?(x=w742, y=u64 1) -> (x = y?=w748:bool)
              n381 = Greater Or Equal?(x=w742, y=u64 2) -> (x >= y?=w754:bool)
              n382 = And(x=w745, y=w730) -> (x .and. y?=w743:bool)
              n383 = And(x=w748, y=w736) -> (x .and. y?=w747:bool)
              n384 = case shown="True" w743 {
                tunnel: w741 -> [_ w779]
                tunnel: w752 -> [_ w780]
                tunnel: w729 -> [_ w770]
                tunnel: [errorcluster {"status"=FALSE, "code"=0, "source"=""} ("error out") w778] -> w726
                tunnel: w725 -> [_ w773]
                tunnel: w724 -> [_ w772]
                tunnel: w722 -> [_ w771]
                frame False {
                }
                frame True {
                  n385 = DataSocket Open(10:T2."Write" ("mode"), 11:w780) -> (0:w784:errorcluster, 3:w783:refnum<k13>)  [unwired: 1 in, 1 out]
                  n386 = DataSocket Write(8:w784, 9:500 ("ms timeout (10000)"), 10:w770, 11:w783) -> (0:w776:errorcluster, 1:w775:bool)  [unwired: 1 out]
                  n387 = Unbundle By Name(w776) -> ("status"=w777:bool)
                  n388 = Or(x=w775, y=w777) -> (x .or. y?=w774:bool)
                  n389 = case shown="False" w774 {
                    tunnel: w779 -> [w799 w816]
                    tunnel: [w798 w814] -> w778
                    tunnel: w773 -> [w795 _]
                    tunnel: w772 -> [w792 _]
                    tunnel: w771 -> [w787 _]
                    tunnel: w770 -> [w791 _]
                    frame False {
                      # "write the actuation instantly."
                      n390 = for {
                        tunnel: w799 -> [w813]
                        tunnel: string[] ["OK! \nActuation is done successfully.", "EndOfTx"] -> [w807] mode=indexing
                        tunnel: [w806] -> w798
                        n391 = String Length(string=w807) -> (length=w811:i32)
                        n392 = Number To Decimal String(number=w811, width (-)=i16 10) -> (decimal integer string=w810:string)
                        n393 = TCP Write(connection ID=w813, data in=w810) -> (connection ID out=w808:refnum<k5>, error out=w809:errorcluster)  [unwired: 2 in, 1 out]
                        n394 = TCP Write(connection ID=w808, data in=w807, error in (no error)=w809) -> (error out=w806:errorcluster)  [unwired: 1 in, 2 out]
                      }
                      n395 = case shown="Default" w787 {
                        tunnel: ["0" "61" "62" "63" "65"] -> w785
                        frame Default {
                        }
                        frame "ST901" {
                        }
                        frame "ST902" {
                        }
                        frame "SV201" {
                        }
                        frame "SV401" {
                        }
                      }
                      n396 = Number To Fractional String(number=w791, precision (6)=i16 2) -> (F-format string=w790:string)  [unwired: 2 in]
                      n397 = Format Date/Time String(time format string (%c)="%y%m%d%H%M%S") -> (date/time string=w793:string)  [unwired: 2 in]
                      n398 = Bundle("2", w785, w787, "A", w790, "date/time string"=w793, "output string"=w792, "0") -> (w796:T4)  [unwired: 1 in]
                      n399 = Enqueue Element(queue=w795, element=w796) -> ()  [unwired: 2 in, 3 out]
                    }
                    frame True {
                      n400 = for {
                        tunnel: w816 -> [w824]
                        tunnel: string[] ["Error in writing the value to the OPC Server!", "EndOfTx"] -> [w818] mode=indexing
                        tunnel: [w817] -> w814
                        n401 = String Length(string=w818) -> (length=w822:i32)
                        n402 = Number To Decimal String(number=w822, width (-)=i16 10) -> (decimal integer string=w821:string)
                        n403 = TCP Write(connection ID=w824, data in=w821) -> (connection ID out=w819:refnum<k5>, error out=w820:errorcluster)  [unwired: 2 in, 1 out]
                        n404 = TCP Write(connection ID=w819, data in=w818, error in (no error)=w820) -> (error out=w817:errorcluster)  [unwired: 1 in, 2 out]
                      }
                    }
                  }
                }
              }
              n405 = case shown="True" w747 {
                tunnel: w741 -> [_ w828]
                tunnel: [errorcluster {"status"=FALSE, "code"=0, "source"=""} ("error out") w826] -> w746
                frame False {
                }
                frame True {
                  n406 = for {
                    tunnel: w828 -> [w836]
                    tunnel: string[] ["Invalid Input!\nData should be between 0 and 100.", "EndOfTx"] -> [w830] mode=indexing
                    tunnel: [w829] -> w826
                    n407 = String Length(string=w830) -> (length=w834:i32)
                    n408 = Number To Decimal String(number=w834, width (-)=i16 10) -> (decimal integer string=w833:string)
                    n409 = TCP Write(connection ID=w836, data in=w833) -> (connection ID out=w831:refnum<k5>, error out=w832:errorcluster)  [unwired: 2 in, 1 out]
                    n410 = TCP Write(connection ID=w831, data in=w830, error in (no error)=w832) -> (error out=w829:errorcluster)  [unwired: 1 in, 2 out]
                  }
                }
              }
              n411 = case shown="True" w754 {
                tunnel: w741 -> [_ w840]
                tunnel: [errorcluster {"status"=FALSE, "code"=0, "source"=""} ("error out") w838] -> w753
                frame False {
                }
                frame True {
                  n412 = for {
                    tunnel: w840 -> [w848]
                    tunnel: string[] ["Invalid Input Parameters!\nMore than One Actuation Found.", "EndOfTx"] -> [w842] mode=indexing
                    tunnel: [w841] -> w838
                    n413 = String Length(string=w842) -> (length=w846:i32)
                    n414 = Number To Decimal String(number=w846, width (-)=i16 10) -> (decimal integer string=w845:string)
                    n415 = TCP Write(connection ID=w848, data in=w845) -> (connection ID out=w843:refnum<k5>, error out=w844:errorcluster)  [unwired: 2 in, 1 out]
                    n416 = TCP Write(connection ID=w843, data in=w842, error in (no error)=w844) -> (error out=w841:errorcluster)  [unwired: 1 in, 2 out]
                  }
                }
              }
              n417 = case shown="True" w758 {
                tunnel: w761 -> [_ w852]
                tunnel: [errorcluster {"status"=FALSE, "code"=0, "source"=""} ("error out") w850] -> w756
                frame False {
                }
                frame True {
                  n418 = for {
                    tunnel: w852 -> [w860]
                    tunnel: string[] ["Invalid Input Parameters!\nNo Actuation Found.", "EndOfTx"] -> [w854] mode=indexing
                    tunnel: [w853] -> w850
                    n419 = String Length(string=w854) -> (length=w858:i32)
                    n420 = Number To Decimal String(number=w858, width (-)=i16 10) -> (decimal integer string=w857:string)
                    n421 = TCP Write(connection ID=w860, data in=w857) -> (connection ID out=w855:refnum<k5>, error out=w856:errorcluster)  [unwired: 2 in, 1 out]
                    n422 = TCP Write(connection ID=w855, data in=w854, error in (no error)=w856) -> (error out=w853:errorcluster)  [unwired: 1 in, 2 out]
                  }
                }
              }
              n423 = Merge Errors(w756, w753, w746, w726) -> (w727:errorcluster)
            }
          }
          n424 = case shown="True" w535 {
            tunnel: w527 -> [_ w968]
            tunnel: w526 -> [_ w967]
            tunnel: w525 -> [_ w966]
            tunnel: w479 -> [_ w962]
            tunnel: [errorcluster {"status"=FALSE, "code"=0, "source"=""} ("error IO") w963] -> w524
            frame False {
            }
            frame True {
              # "check each row of the array to see if it matches. If yes, append that row to the result array"
              n425 = local read "Real-time Data from Motes"() -> (w969:string[][])
              n426 = for {
                tunnel: w969 -> [w995] mode=indexing
                tunnel: w968 -> [w997]
                tunnel: w967 -> [w1002]
                tunnel: w966 -> [w1001]
                shift-right: [w999] -> w964
                shift-left: string[][] [] -> [w996]
                i -> [w994]
                stop <- TRUE continue-if-true
                n427 = case shown="Default" w994 {
                  tunnel: w1002 -> [_ w1015]
                  tunnel: w1001 -> [_ w1014]
                  tunnel: [TRUE w1013] -> w1000
                  tunnel: w997 -> [_ w1012]
                  tunnel: w995 -> [_ w1011]
                  tunnel: w995 -> [_ w1004]
                  frame 0 {
                  }
                  frame Default {
                    n428 = Index Array(array=w1011, index=1) -> (element=w1009:string)
                    n429 = Empty String/Path?(string/path=w1012) -> (empty?=w1007:bool)
                    n430 = Equal?(x=w1012, y=w1009) -> (x = y?=w1008:bool)
                    n431 = Or(x=w1007, y=w1008) -> (x .or. y?=w1006:bool)
                    n432 = case shown="True" w1006 {
                      tunnel: w1011 -> [_ w1030]
                      tunnel: w1015 -> [_ w1025]
                      tunnel: [FALSE w1028] -> w1005
                      frame False {
                      }
                      frame True {
                        n433 = Index Array(array=w1030, index=2) -> (element=w1029:string)
                        n434 = Empty String/Path?(string/path=w1025) -> (empty?=w1026:bool)
                        n435 = Equal?(x=w1025, y=w1029) -> (x = y?=w1027:bool)
                        n436 = Or(x=w1026, y=w1027) -> (x .or. y?=w1028:bool)
                      }
                    }
                    n437 = case shown="True" w1005 {
                      tunnel: w1004 -> [_ w1022]
                      tunnel: w1014 -> [_ w1018]
                      tunnel: [FALSE w1017] -> w1013
                      frame False {
                      }
                      frame True {
                        n438 = Index Array(array=w1022, index=3) -> (element=w1021:string)
                        n439 = Equal?(x=w1018, y=w1021) -> (x = y?=w1020:bool)
                        n440 = Empty String/Path?(string/path=w1018) -> (empty?=w1019:bool)
                        n441 = Or(x=w1019, y=w1020) -> (x .or. y?=w1017:bool)
                      }
                    }
                  }
                }
                n442 = case shown="True" w1000 {
                  tunnel: w996 -> [w1032 w1035]
                  tunnel: w995 -> [_ w1034]
                  tunnel: [w1032 w1033] -> w999
                  frame False {
                  }
                  frame True {
                    n443 = Build Array (concatenate)(w1035, w1034) -> (w1033:string[][])
                  }
                }
              }
              n444 = flat-sequence {
                tunnel: w964 -> [w972]
                tunnel: w962 -> [w971]
                tunnel: [w970] -> w961
                tunnel: [w984] -> w963
                tunnel: w962 -> [w986]
                tunnel: w961 -> [w985]
                frame #0 {
                  # "send each element of the array through the TCP connection"
                  n445 = for {
                    tunnel: w972 -> [w975] mode=indexing
                    tunnel: w971 -> [w974]
                    tunnel: [w973] -> w970
                    n446 = for {
                      tunnel: w975 -> [w978] mode=indexing
                      tunnel: w974 -> [w977]
                      tunnel: [w976] -> w973
                      n447 = String Length(string=w978) -> (length=w982:i32)
                      n448 = Number To Decimal String(number=w982, width (-)=i16 10) -> (decimal integer string=w981:string)
                      n449 = TCP Write(connection ID=w977, data in=w981) -> (connection ID out=w979:refnum<k5>, error out=w980:errorcluster)  [unwired: 2 in, 1 out]
                      n450 = TCP Write(connection ID=w979, data in=w978, error in (no error)=w980) -> (error out=w976:errorcluster)  [unwired: 1 in, 2 out]
                    }
                  }
                }
                frame #1 {
                  w988 = "EndOfTx" ("data in")
                  n451 = String Length(string=w988) -> (length=w991:i32)
                  n452 = Number To Decimal String(number=w991, width (-)=i16 10) -> (decimal integer string=w992:string)
                  n453 = TCP Write(connection ID=w986, data in=w992) -> (connection ID out=w989:refnum<k5>, error out=w993:errorcluster)  [unwired: 2 in, 1 out]
                  n454 = TCP Write(connection ID=w989, data in=w988, error in (no error)=w993) -> (error out=w987:errorcluster)  [unwired: 1 in, 2 out]
                  n455 = Merge Errors(w987, w985) -> (w984:errorcluster)
                }
              }
            }
          }
          n456 = Merge Errors(w524, w523, w515, w505, w494, w477, w478) -> (w529:errorcluster)
          "Req / Res Error" <- w529
          n457 = Unbundle By Name(w529) -> ("status"=w473:bool)
          n458 = Or(x="stop", y=w473) -> (x .or. y?=w475:bool)
        }
      }
      frame Error {
      }
    }
  }
